vi "Tilted Logistic Square Pulse Fit Result String.vi"(8 "error in (no error)":errorcluster, 9 "Delta Best Fit Parameters":dbl[](array[numeric]), 10 "Fit Output":T1={"best nonlinear fit"=[], "best fit parameters"=[], "R^2"=0.0, "RMSE"=0.0, "error out"={"status"=FALSE, "code"=0, "source"=""}, "Fitting Method"=enum."Least Square", "number of function calls"=0, "number of iterations"=0, "covariance"=[], "Chi 2"=0.0, "DOF"=0, "Fit Convergence Criterion"=enum."Continue", "Fitting Algorithm"=enum."Levenberg-Marquardt", "Weighted Fit"=enum."Unweighted", "Gradient"=0.0, "|Delta Chi 2|"=0.0, "|Delta Chi 2|/Chi 2"=0.0, "Max |Delta a| /|a|"=0.0, "Lambda"=-1.0, "RSS"=0.0, "AIC"=0.0, "BIC"=0.0, "Max number of function calls"=0, "Max number of iterations"=0, "IRF"={"X Array"=[], "Y Array"=[]}, "IRF Normalization Factor"=0.0, "Decay Normalization Factor"=0.0, "Number of offset fits"=0, "Weighted Chi2"=-1.0, "Unweighted Chi2"=-1.0}, 11 "ROI Descriptor":T8 {"Contours"."Type" items=["No Selection", "Point", "Line", "Rectangle", "Oval", "Polygon", "Freehand Region", "Annulus", "Unused2", "Unused3", "Broken Line", "Freehand Line", "Rotated Rectangle"]}) -> (0 "error out":errorcluster, 3 "Result String":string)   [LabVIEW 2021, in "Fits.lvlib"]
uses:
  Fits.lvlib
  Non-linear Fit Output v4.ctl
  Nonlinear Fit Method.ctl
  <vilib>/Analysis/Matrix/Datatypes/RealMatrix.ctl
  Convergence Criteria.ctl
  Non-linear Fitting Algorithm.ctl
  IRF(X)PSED/Fit Weights Type v2.ctl
  Graphs/XY Graph/XY Graph Plot Data.ctl
  <vilib>/Analysis/Matrix/NI_Matrix.lvlib
  Graphs/XY Graph/XY Graph Add-Ons.lvlib
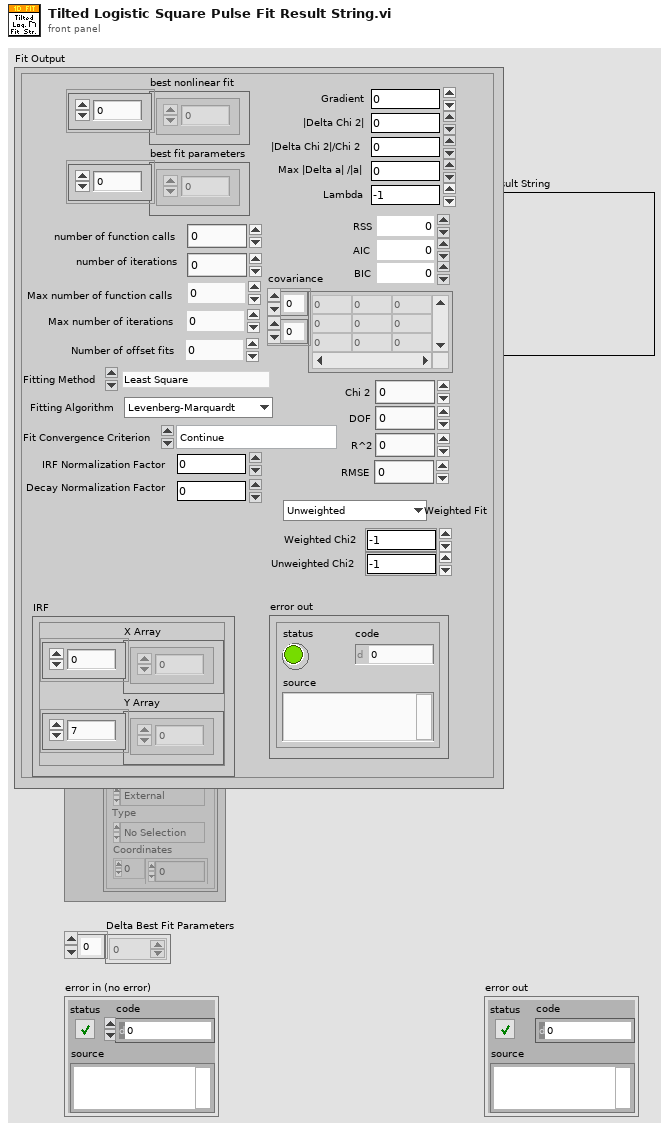
[diagram p1: front panel]
types:
  T1 = typedef "Fits.lvlib/Non-linear Fit Output v4.ctl" = cluster{"best nonlinear fit":dbl[], "best fit parameters":dbl[], "R^2":dbl, "RMSE":dbl, "error out":errorcluster, "Fitting Method":T2, "number of function calls":i32, "number of iterations":i32, "covariance":T3, "Chi 2":dbl, "DOF":i32, "Fit Convergence Criterion":T4, "Fitting Algorithm":T5, "Weighted Fit":T6, "Gradient":dbl, "|Delta Chi 2|":dbl, "|Delta Chi 2|/Chi 2":dbl, "Max |Delta a| /|a|":dbl, "Lambda":dbl, "RSS":dbl, "AIC":dbl, "BIC":dbl, "Max number of function calls":i32, "Max number of iterations":i32, "IRF":T7, "IRF Normalization Factor":dbl, "Decay Normalization Factor":dbl, "Number of offset fits":i32, "Weighted Chi2":dbl, "Unweighted Chi2":dbl}
  T2 = typedef "Fits.lvlib/Nonlinear Fit Method.ctl" = enum16{"Least Square", "Least Absolute Residual", "Bisquare", "MLE"}
  T3 = typedef "NI_Matrix.lvlib/RealMatrix.ctl" = dbl[][]
  T4 = typedef "Fits.lvlib/Convergence Criteria.ctl" = enum16{"Continue", "Tolerances Exceeded", "Max Time Exceeded", "Max Iterations Exceeded", "Max Function Evaluations Exceeded", "Scale Range Exceeded"}
  T5 = typedef "Fits.lvlib/Non-linear Fitting Algorithm.ctl" = enum16{"Levenberg-Marquardt", "Trust-Region Dogleg"}
  T6 = typedef "Fits.lvlib/Fit Weights Type v2.ctl" = enum16{"Unweighted", "1/Variance (Neyman)", "1/Variance (Pearson)", "Best of All"}
  T7 = typedef "XY Graph Add-Ons.lvlib/XY Graph Plot Data.ctl" = cluster{"X Array":dbl[], "Y Array":dbl[]}
  T8 = typedef "ROI Descriptor" = cluster{"Global Rectangle":i32[], "Contours":cluster{"ID":enum32{"External", "Internal"}, "Type":u32, "Coordinates":i32[]}[]}
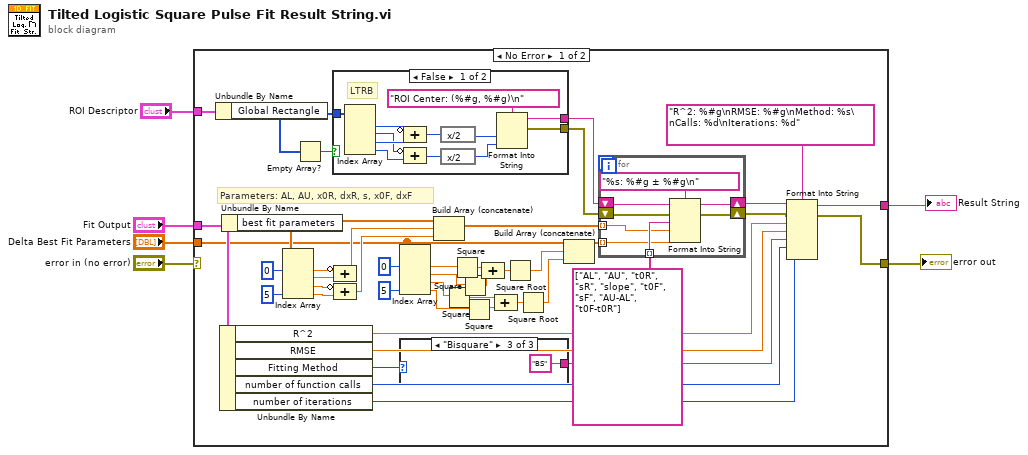
[diagram p0: block diagram]
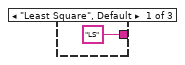
[diagram p3: hidden frame]
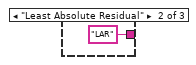
[diagram p4: hidden frame]
diagram:
  n1 = case shown="No Error" "error in (no error)" {
    selector: "error in (no error)" -> [_ w74]
    tunnel: [w42 w74] -> w5
    tunnel: "ROI Descriptor" -> [w50 _]
    tunnel: "Fit Output" -> [w47 _]
    tunnel: "Delta Best Fit Parameters" -> [w11 _]
    tunnel: [w43 _] -> w1
    frame No Error {
      # "Parameters: AL, AU, x0R, dxR, s, x0F, dxF"
      n2 = Unbundle By Name(w50) -> ("Global Rectangle"=w35:i32[])
      n3 = Unbundle By Name(w47) -> ("R^2"=w41:dbl, "RMSE"=w40:dbl, "Fitting Method"=w39:T2, "number of function calls"=w37:i32, "number of iterations"=w36:i32)
      n4 = Unbundle By Name(w47) -> ("best fit parameters"=w32:dbl[])
      n5 = Index Array(array=w32, index #1=0 ("index"), index #4=5 ("index")) -> (element #1=w22:dbl, element #2=w21:dbl, element #3=w20:dbl, element #4=w19:dbl)  [unwired: 2 in]
      n6 = Empty Array?(array=w35) -> (empty?=w34:bool)
      n7 = case shown="False" w34 {
        tunnel: [w53 _] -> w49
        tunnel: [w52 _] -> w48
        tunnel: w35 -> [w51 _]
        frame False {
          # "LTRB"
          n8 = Index Array(array=w51) -> (element #1=w62:i32, element #2=w59:i32, element #3=w61:i32, element #4=w60:i32)  [unwired: 4 in]
          n9 = Compound Arithmetic op=ADD(invert w62, w61) -> (w58:i32)
          n10 = Compound Arithmetic op=ADD(invert w59, w60) -> (w57:i32)
          n11 = expression code="x/2"(w58) -> (w55:i32)
          n12 = expression code="x/2"(w57) -> (w54:i32)
          n13 = Format Into String(format string="ROI Center: (%#g, %#g)\n", w55, w54) -> (resulting string=w52:string, error out=w53:errorcluster)  [unwired: 2 in]
        }
        frame True {
        }
      }
      n14 = Compound Arithmetic op=ADD(invert w22, w21) -> (w28:dbl)
      n15 = Compound Arithmetic op=ADD(invert w20, w19) -> (w24:dbl)
      n16 = Index Array(array=w11, index #1=0 ("index"), index #4=5 ("index")) -> (element #1=w10:dbl, element #2=w9:dbl, element #3=w8:dbl, element #4=w7:dbl)  [unwired: 2 in]
      n17 = case shown="\"Bisquare\"" w39 {
        tunnel: ["LS" ("input 3") "LAR" ("input 3") "BS" ("input 3")] -> w38
        frame "Least Square", Default {
        }
        frame "Least Absolute Residual" {
        }
        frame "Bisquare" {
        }
      }
      n18 = Build Array (concatenate)(w32, w28, w24) -> (w29:dbl[])
      n19 = Square(x=w8) -> (x^2=w17:dbl)
      n20 = Square(x=w10) -> (x^2=w27:dbl)
      n21 = Square(x=w9) -> (x^2=w26:dbl)
      n22 = Square(x=w7) -> (x^2=w16:dbl)
      n23 = Compound Arithmetic op=ADD(w27, w26) -> (w25:dbl)
      n24 = Compound Arithmetic op=ADD(w17, w16) -> (w18:dbl)
      n25 = Square Root(x=w25) -> (sqrt(x)=w15:dbl)
      n26 = Square Root(x=w18) -> (sqrt(x)=w14:dbl)
      n27 = Build Array (concatenate)(w11, w15, w14) -> (w23:dbl[])
      n28 = for {
        tunnel: w29 -> [w66] mode=indexing
        tunnel: w23 -> [w67] mode=indexing
        shift-right: [w71] -> w46
        shift-left: w48 -> [w72]
        shift-right: [w70] -> w45
        shift-left: w49 -> [w69]
        tunnel: string[] ["AL", "AU", "t0R", "sR", "slope", "t0F", "sF", "AU-AL", "t0F-t0R"] -> [w68] mode=indexing
        n29 = Format Into String(format string="%s: %#g ± %#g\n", initial string=w72, error in=w69, w68, w66, w67) -> (resulting string=w71:string, error out=w70:errorcluster)
      }
      n30 = Format Into String(format string="R^2: %#g\nRMSE: %#g\nMethod: %s\nCalls: %d\nIterations: %d", initial string=w46, error in=w45, w41, w40, w38, w37, w36) -> (resulting string=w43:string, error out=w42:errorcluster)
    }
    frame Error {
    }
  }
  "Result String" <- w1
  "error out" <- w5
